vi "front Sw--L.vi"(8 "Command Info In":T1, 10 "F-SW--Line":T4, 11 "Switch":string) -> (0 "Command Info Out":T1)   [LabVIEW 2017]
uses:
  Block Clusters/front Sw--L.ctl
  <vilib>/Rock Robotics/WPI/Framework/Command Status Info.ctl
  <vilib>/Rock Robotics/WPI/Framework/Completion Status.ctl
  <vilib>/Rock Robotics/WPI/Framework/Completion Notifier.ctl
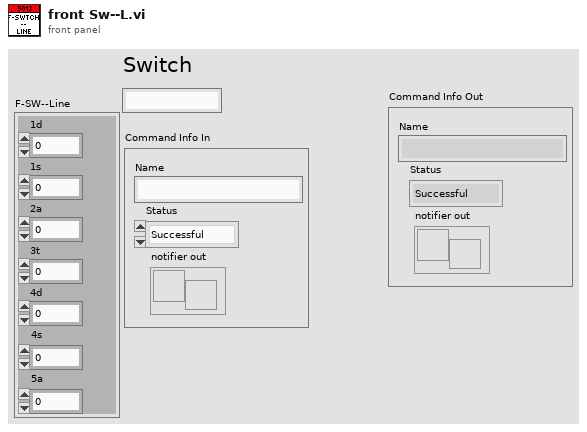
[diagram p1: front panel]
types:
  T1 = typedef "Command Status Info.ctl" = cluster{"Name":string, "Status":T2, "notifier out":T3}
  T2 = typedef "Completion Status.ctl" = enum16{"Successful", "Aborted", "Incomplete"}
  T3 = typedef "Completion Notifier.ctl" = refnum<notifier>
  T4 = typedef "front Sw--L.ctl" = cluster{"1d":dbl, "1s":dbl, "2a":dbl, "3t":dbl, "4d":dbl, "4s":dbl, "5a":dbl}
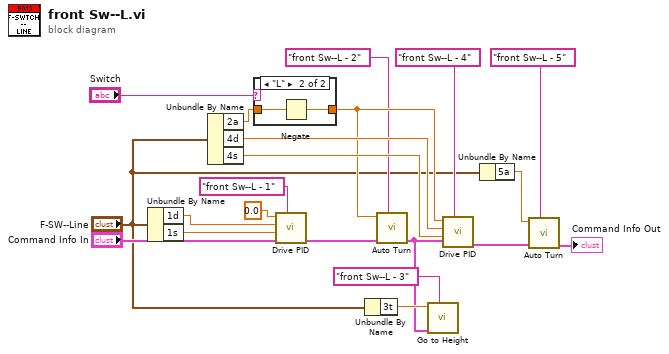
[diagram p0: block diagram]
diagram:
  n1 = Unbundle By Name("F-SW--Line") -> ("1d"=w21:dbl, "1s"=w20:dbl)
  n2 = Unbundle By Name("F-SW--Line") -> ("2a"=w13:dbl, "4d"=w17:dbl, "4s"=w16:dbl)
  n3 = case shown="\"L\"" "Switch" {
    tunnel: w13 -> [w22 w24]
    tunnel: [w22 w23] -> w12
    frame "R", Default {
    }
    frame "L" {
      n4 = Negate(x=w24) -> (-x=w23:dbl)
    }
  }
  n5 = call "Drive PID.vi"("Description"="front Sw--L - 1", "Command Info In"="Command Info In", "Speed"=w20, "Distance"=w21, "Target Angle"=0.0) -> ("Command Info Out"=w18:T1)  [unwired: 6 in]
  n6 = Unbundle By Name("F-SW--Line") -> ("3t"=w9:dbl)
  n7 = call "Auto Turn.vi"("Description"="front Sw--L - 2", "Command Info In"=w18, "Target Angle"=w12) -> ("Command Info Out"=w8:T1)  [unwired: 8 in]
  n8 = call "Go to Height.vi"("Description"="front Sw--L - 3", "Command Info In"=w8, "Target Height (in)"=w9) -> ()  [unwired: 8 in, 1 out]
  n9 = call "Drive PID.vi"("Description"="front Sw--L - 4", "Command Info In"=w8, "Speed"=w16, "Distance"=w17, "Target Angle"=w12) -> ("Command Info Out"=w15:T1)  [unwired: 6 in]
  n10 = Unbundle By Name("F-SW--Line") -> ("5a"=w3:dbl)
  n11 = call "Auto Turn.vi"("Description"="front Sw--L - 5", "Command Info In"=w15, "Target Angle"=w3) -> ("Command Info Out"=→"Command Info Out":T1)  [unwired: 8 in]
